vi "Set Number of Cameras.vi"(8 "error in (no error)":errorcluster, 10 "Cameras":i32, 11 "Main Window in":refnum<class "Main Window.lvclass">) -> (0 "error out":errorcluster, 3 "Main Window out":refnum<class "Main Window.lvclass">)   [LabVIEW 2015, in "Main Window.lvlib" / "Main Window.lvclass"]
uses:
  Main Window.lvclass
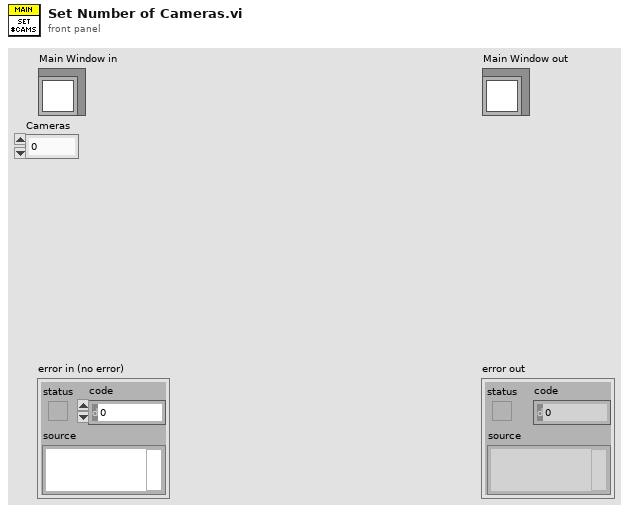
[diagram p1: front panel]
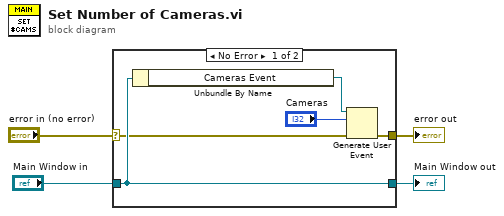
[diagram p0: block diagram]
diagram:
  n1 = case shown="No Error" "error in (no error)" {
    selector: "error in (no error)" -> [w6 w11]
    tunnel: [w5 w11] -> w3
    tunnel: [w9 w10] -> w1
    tunnel: "Main Window in" -> [w9 w10]
    frame No Error {
      n2 = Unbundle By Name(w9) -> ("Cameras Event"=w8:refnum<user-event>)
      n3 = Generate User Event(user event=w8, event data cluster="Cameras", error in=w6) -> (error out=w5:errorcluster)  [unwired: 1 in, 1 out]
    }
    frame Error {
    }
  }
  "error out" <- w3
  "Main Window out" <- w1
